vi "PC Main.vi"() -> ()   [LabVIEW 2018]
uses:
  <vilib>/Math Plots/2D Math Plots/2D Error Bar/2D Error Bar XCtrl/2D Error Bar.xctl
panel:
  out "last count":bool
  in  "Count":u32
  in  "Tab Control":enum32{"Page 1", "Page 2"}(tab)
  in  "Sample rate (Ticks) 2":i64
  in  "Sample rate (Ticks) 1":i64
  in  "Lower Threshold 2":i64
  in  "Lower Threshold 1":i64
  in  "OK Button":bool
  in  "Clockwise":bool
  in  "Asix":u32
  in  "?":bool
  in  "Gated 1 (us)":i32
  in  "Gated 2 (us)":i32
  in  "Delay 1 (us)":i32
  in  "Delay 2 (us)":i32
  in  "Boolean 2":bool
  in  "Time Step":u32
  out "Current count":u32
  in  "?":bool
  in  "Step Angle":u32
  out "initialized array":dbl[][](array[numeric])
  in  "Max":u32
  in  "Min":u32
  out "Current Angle":u32
  out "2D Error Bar 2":refnum<class "2D Plot Datatype.lvclass">[](xcontrol)
  out "Time (s)":string
  # "Counter-Clockwise"
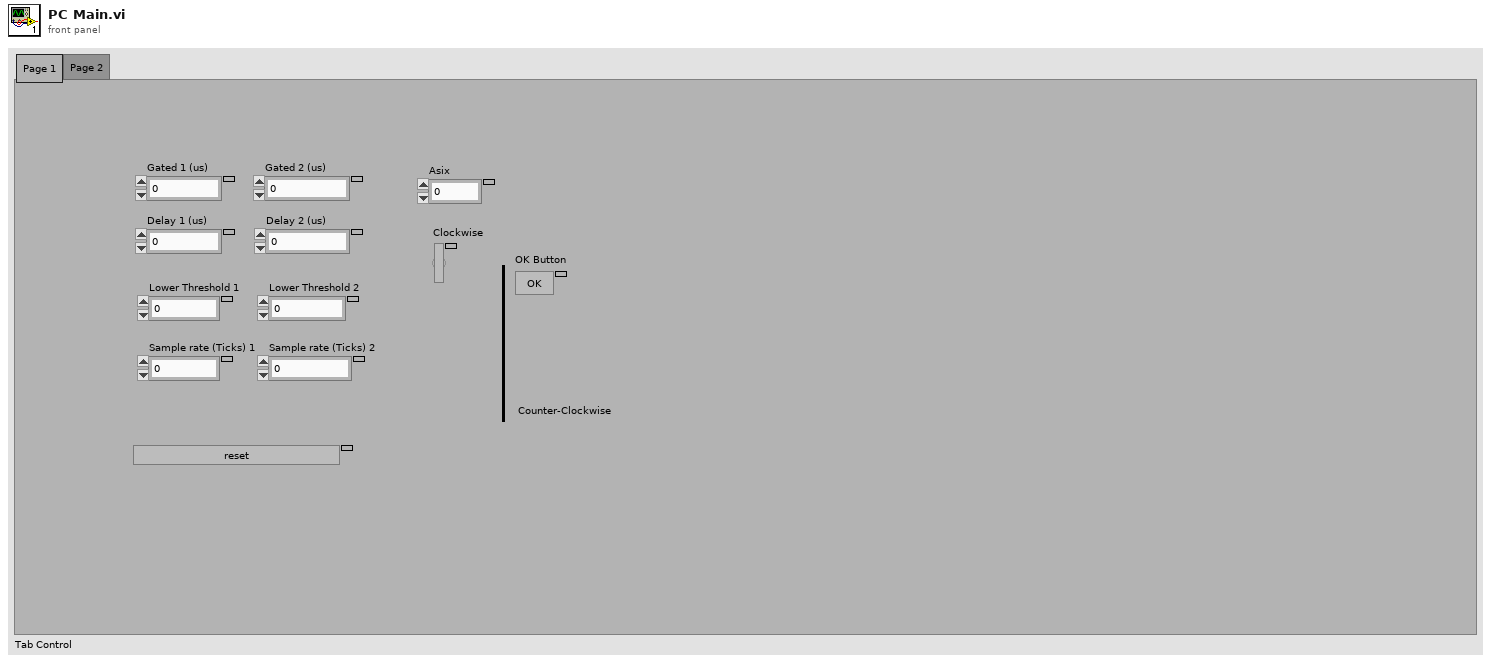
[diagram p1: front panel]
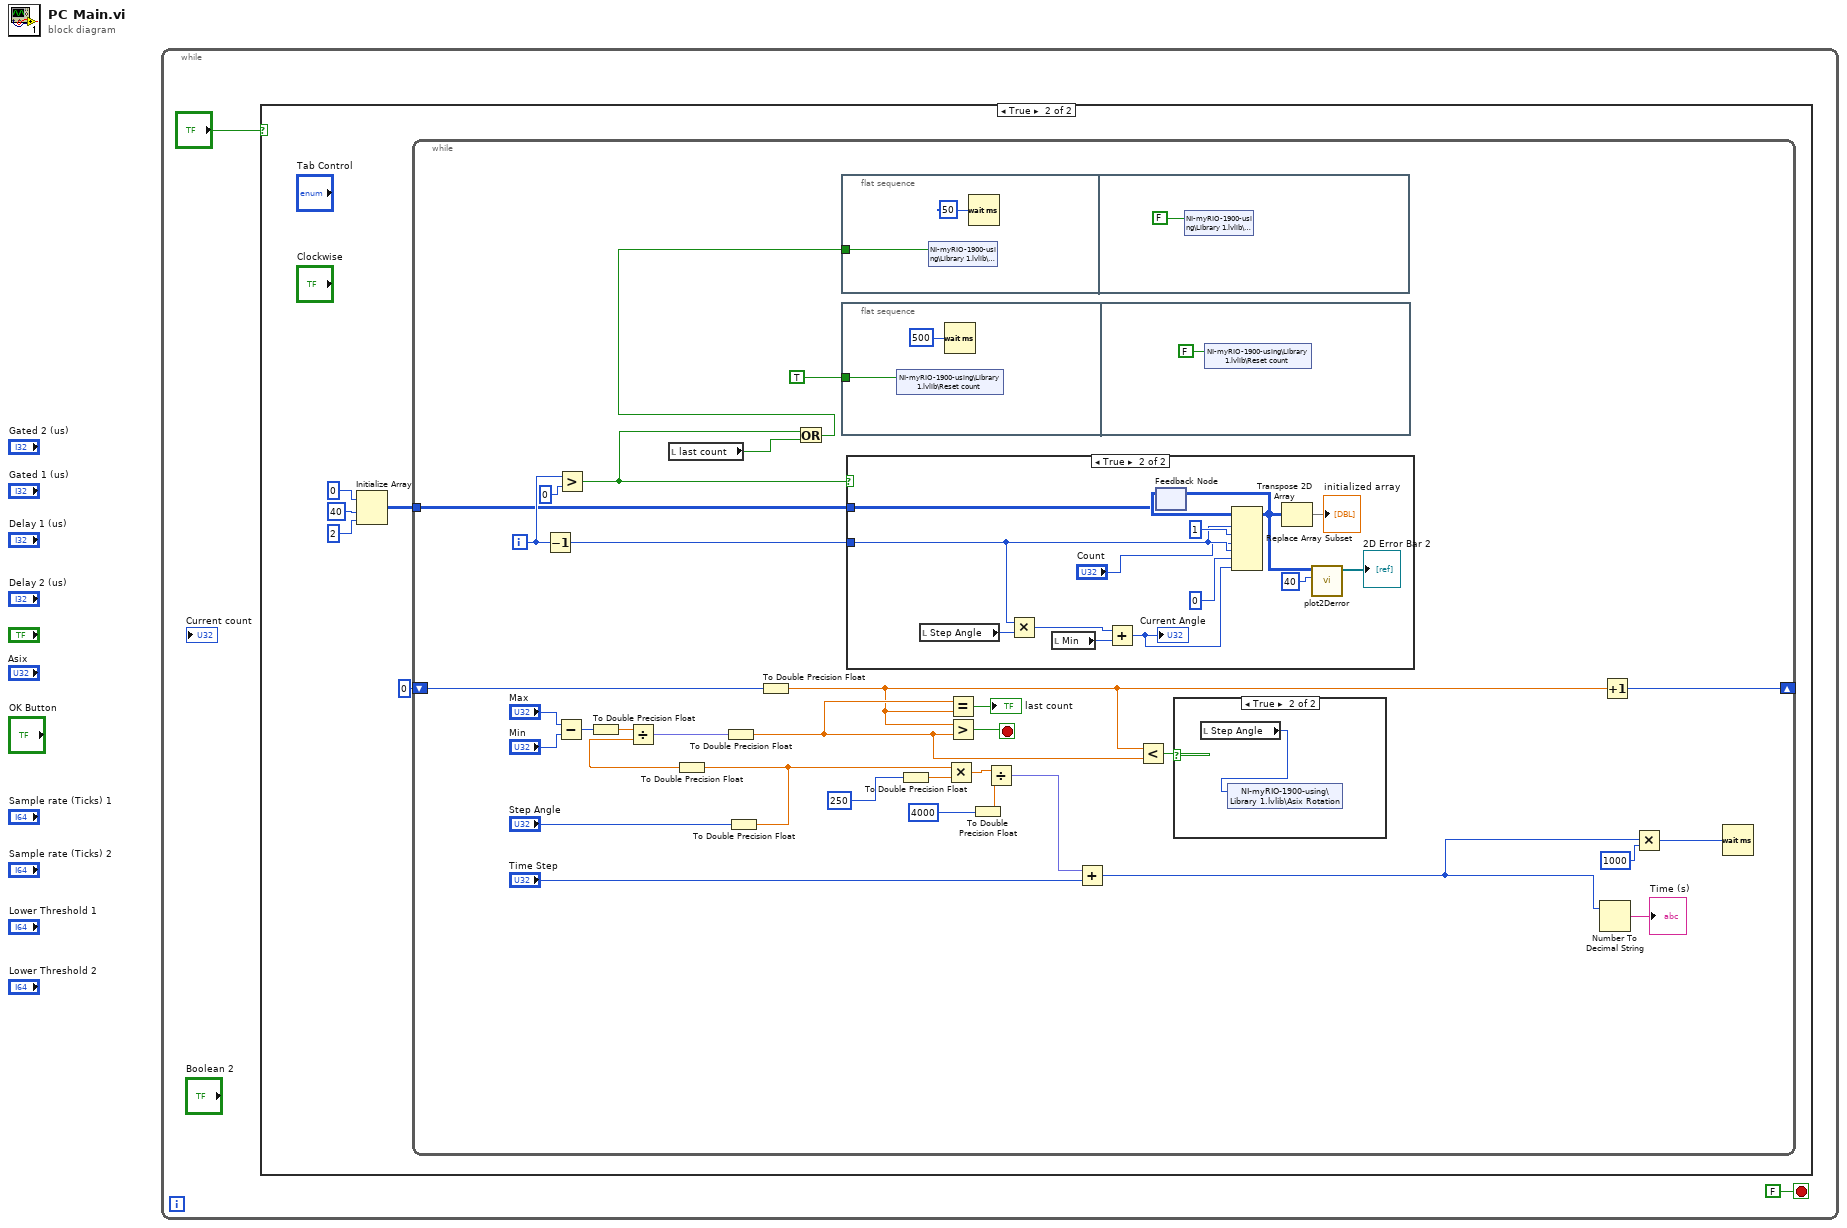
[diagram p0: block diagram]
diagram:
  n1 = while {
    stop <- FALSE stop-if-true
    n2 = case shown="True" "?" {
      frame False {
      }
      frame True {
        n3 = Initialize Array(0 ("element"), 40 ("dimension size"), 2 ("dimension size")) -> (w3:i32[][])
        n4 = while {
          shift-right: [w36] -> _
          shift-left: 0 -> [w15]
          tunnel: w3 -> [w12]
          i -> [w32]
          stop <- w17 stop-if-true
          n5 = Decrement(x=w32) -> (x-1=w16:i32)
          n6 = Subtract(x="Max", y="Min") -> (x-y=w26:u32)
          n7 = Greater?(x=w32, y=0) -> (0:w30:bool)
          n8 = To Double Precision Float(number=w26) -> (double precision float=w23:dbl)
          n9 = local read "last count"() -> (w29:bool)
          n10 = To Double Precision Float(number="Step Angle") -> (double precision float=w22:dbl)
          n11 = To Double Precision Float(number=w22) -> (double precision float=w21:dbl)
          n12 = Divide(x=w23, y=w21) -> (x/y=w25:fxp<+,32,16>)
          n13 = To Double Precision Float(number=w25) -> (double precision float=w24:dbl)
          n14 = To Double Precision Float(number=w15) -> (double precision float=w19:dbl)
          n15 = Or(x=w30, y=w29) -> (x .or. y?=w28:bool)
          n16 = flat-sequence {
            tunnel: w28 -> [w60]
            frame #0 {
              n17 = shared-variable "NI-myRIO-1900-using\\Library 1.lvlib\\Start"(w60) -> ()  [unwired: 1 in, 1 out]
              n18 = Wait (ms)(milliseconds to wait=u32 50) -> ()  [unwired: 1 out]
            }
            frame #1 {
              n19 = shared-variable "NI-myRIO-1900-using\\Library 1.lvlib\\Start"(FALSE ("Reset count")) -> ()  [unwired: 1 in, 1 out]
            }
          }
          n20 = flat-sequence {
            tunnel: TRUE -> [w57]
            frame #0 {
              n21 = shared-variable "NI-myRIO-1900-using\\Library 1.lvlib\\Reset count"(w57) -> ()  [unwired: 1 in, 1 out]
              n22 = Wait (ms)(milliseconds to wait=u32 500) -> ()  [unwired: 1 out]
            }
            frame #1 {
              n23 = shared-variable "NI-myRIO-1900-using\\Library 1.lvlib\\Reset count"(FALSE) -> ()  [unwired: 1 in, 1 out]
            }
          }
          n24 = case shown="True" w30 {
            tunnel: w12 -> [_ w49]
            tunnel: w16 -> [_ w45]
            frame False {
            }
            frame True {
              n25 = local read "Step Angle"() -> (w51:u32)
              n26 = Multiply(x=w45, y=w51) -> (x*y=w52:u32)
              n27 = local read "Min"() -> (w46:u32)
              n28 = Add(x=w52, y=w46) -> (x+y=w44:u32)
              "Current Angle" <- w44
              n29 = feedback #1(w49) -> (w53:i32[][])
              n30 = Replace Array Subset(array=w53, new element #1="Count", index (row) #1=w45, index (col) #1=1 ("disabled index (col)"), new element #2=w44, index (row) #2=w45, index (col) #2=0 ("index (col)")) -> (w55:i32[][])
              n31 = feedback-in #1(w55) -> ()
              n32 = Transpose 2D Array(2D array=w55) -> (transposed array=→"initialized array":i32[][])
              n33 = call "plot2Derror.vi"("length"=40, "2D array"=w55) -> ("2D Error Bar"=→"2D Error Bar 2":refnum<class "2D Plot Datatype.lvclass">[])  [unwired: 9 in]
            }
          }
          n34 = To Double Precision Float(number=u32 250 ("y")) -> (double precision float=w20:dbl)
          n35 = Multiply(x=w22, y=w20) -> (x*y=w40:dbl)
          n36 = Equal?(x=w24, y=w19) -> (x = y?=→"last count":bool)
          n37 = Greater?(x=w19, y=w24) -> (0:w17:bool)
          n38 = To Double Precision Float(number=u32 4000 ("y")) -> (double precision float=w18:dbl)
          n39 = Divide(x=w40, y=w18) -> (x/y=w39:fxp<+,32,16>)
          n40 = Add(x=w39, y="Time Step") -> (x+y=w8:i64)
          n41 = Less?(x=w19, y=w24) -> (x < y?=w9:bool)
          n42 = case shown="True" w9 {
            frame False {
            }
            frame True {
              n43 = local read "Step Angle"() -> (w42:u32)
              n44 = shared-variable "NI-myRIO-1900-using\\Library 1.lvlib\\Asix Rotation"(w42) -> ()  [unwired: 1 in, 1 out]
            }
          }
          n45 = Number To Decimal String(number=w8) -> (decimal integer string=→"Time (s)":string)  [unwired: 1 in]
          n46 = Increment(x=w19) -> (x+1=w36:i32)
          n47 = Multiply(x=w8, y=i64 1000) -> (x*y=w38:i64)
          n48 = Wait (ms)(milliseconds to wait=w38) -> ()  [unwired: 1 out]
        }
      }
    }
  }
